vi "List Mode - Set Configurations for Sequence Setup.vi"   [LabVIEW 2014, in "Associated Power Technologies 8500 Series.lvlib"]
uses:
  <instrlib>/Associated Power Technologies 8500 Series/Associated Power Technologies 8500 Series.lvlib
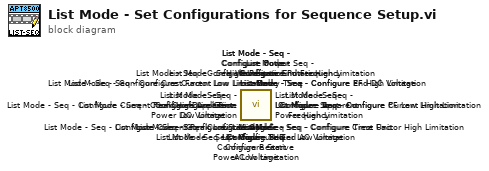
[diagram p0: block diagram]
diagram:
  n1 = call <instrlib>:"List Mode - Seq - Configure THD.vi"() -> ()  [unwired: 10 in, 2 out]
  n2 = call <instrlib>:"List Mode - Seq - Configure Limitation Delay Time.vi"() -> ()  [unwired: 10 in, 2 out]
  n3 = call <instrlib>:"List Mode - Seq - Configure Apparent Power Low Limitation.vi"() -> ()  [unwired: 10 in, 2 out]
  n4 = call <instrlib>:"List Mode - Seq - Configure Apparent Power High Limitation.vi"() -> ()  [unwired: 10 in, 2 out]
  n5 = call <instrlib>:"List Mode - Seq - Configure Crest Factor Low Limitation.vi"() -> ()  [unwired: 10 in, 2 out]
  n6 = call <instrlib>:"List Mode - Seq - Configure Crest Factor High Limitation.vi"() -> ()  [unwired: 10 in, 2 out]
  n7 = call <instrlib>:"List Mode - Seq - Configure Reactive Power Low Limitation.vi"() -> ()  [unwired: 10 in, 2 out]
  n8 = call <instrlib>:"List Mode - Seq - Configure Reactive Power High Limitation.vi"() -> ()  [unwired: 10 in, 2 out]
  n9 = call <instrlib>:"List Mode - Seq - Configure Current Peak Low Limitation.vi"() -> ()  [unwired: 10 in, 2 out]
  n10 = call <instrlib>:"List Mode - Seq - Configure Current Peak High Limitation.vi"() -> ()  [unwired: 10 in, 2 out]
  n11 = call <instrlib>:"List Mode - Seq - Configure PF Low Limitation.vi"() -> ()  [unwired: 10 in, 2 out]
  n12 = call <instrlib>:"List Mode - Seq - Configure PF High Limitation.vi"() -> ()  [unwired: 10 in, 2 out]
  n13 = call <instrlib>:"List Mode - Seq - Configure Power Low Limitation.vi"() -> ()  [unwired: 10 in, 2 out]
  n14 = call <instrlib>:"List Mode - Seq - Configure Power High Limitation.vi"() -> ()  [unwired: 10 in, 2 out]
  n15 = call <instrlib>:"List Mode - Seq - Configure Current Low Limitation.vi"() -> ()  [unwired: 10 in, 2 out]
  n16 = call <instrlib>:"List Mode - Seq - Configure Current High Limitation.vi"() -> ()  [unwired: 10 in, 2 out]
  n17 = call <instrlib>:"List Mode - Seq - Configure Time Unit.vi"() -> ()  [unwired: 10 in, 2 out]
  n18 = call <instrlib>:"List Mode - Seq - Configure Dwell Time.vi"() -> ()  [unwired: 10 in, 2 out]
  n19 = call <instrlib>:"List Mode - Seq - Configure Cycle.vi"() -> ()  [unwired: 10 in, 2 out]
  n20 = call <instrlib>:"List Mode - Seq - Configure End DC Voltage.vi"() -> ()  [unwired: 10 in, 2 out]
  n21 = call <instrlib>:"List Mode - Seq - Configure End Frequency.vi"() -> ()  [unwired: 10 in, 2 out]
  n22 = call <instrlib>:"List Mode - Seq - Configure End AC Voltage.vi"() -> ()  [unwired: 10 in, 2 out]
  n23 = call <instrlib>:"List Mode - Seq - Configure Start DC Voltage.vi"() -> ()  [unwired: 10 in, 2 out]
  n24 = call <instrlib>:"List Mode - Seq - Configure Start Frequency.vi"() -> ()  [unwired: 10 in, 2 out]
  n25 = call <instrlib>:"List Mode - Seq - Configure Start AC Voltage.vi"() -> ()  [unwired: 10 in, 2 out]
  n26 = call <instrlib>:"List Mode - Seq - Configure Start Angle.vi"() -> ()  [unwired: 10 in, 2 out]
  n27 = call <instrlib>:"List Mode - Seq - Configure Output Waveform.vi"() -> ()  [unwired: 10 in, 2 out]
